vi "grafica.vi"() -> ()   [LabVIEW 2025]
panel:
  in  "stop":bool
  out "Waveform Graph":dbl[](graph)
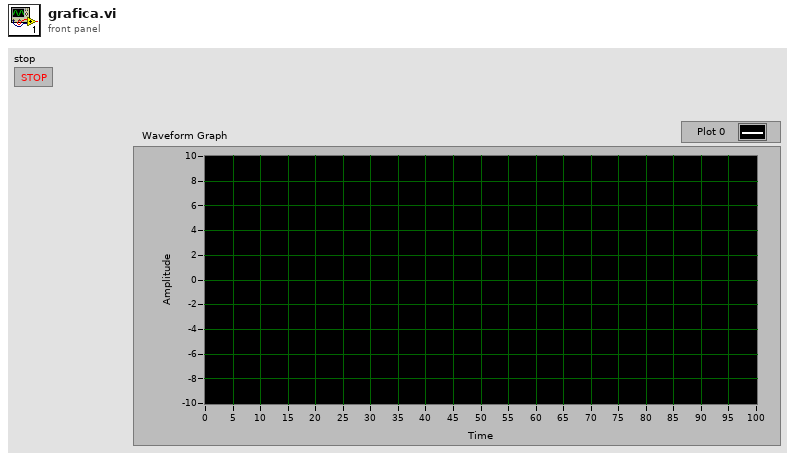
[diagram p1: front panel]
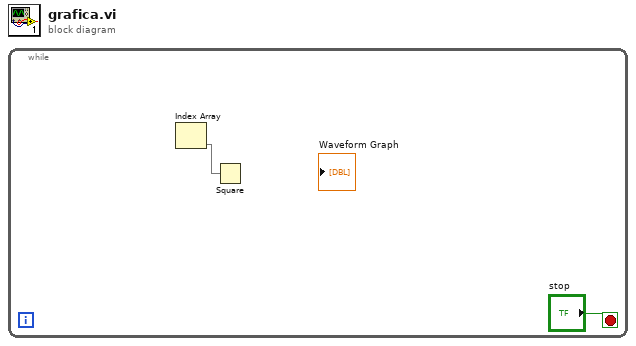
[diagram p0: block diagram]
diagram:
  n1 = while {
    stop <- "stop" stop-if-true
    n2 = Index Array() -> (element=w1)  [unwired: 2 in]
    n3 = Square(x=w1) -> ()  [unwired: 1 out]
  }
